vi "Insert While Loop.vi"(6 "Insertion Index":i32=-1, 7 "Parent ID":string, 8 "error in (no error)":errorcluster, 9 "Unique ID":string, 10 "Name":string, 11 "Test Executive Ref":refnum<data-value>) -> (0 "error out":errorcluster, 1 "Replaced?":bool, 3 "Test Executive Ref out":refnum<data-value>, 5 "Unique ID out":string)   [LabVIEW 2017, in "Test Executive.lvlib" / "TestExecutive Ref.lvclass"]
uses:
  <vilib>/gpm_packages/@cs/test-executive/Source/Test Executive/TestExecutive Ref/TestExecutive Ref.lvclass
  <vilib>/gpm_packages/@cs/test-executive/Source/Test Executive/ITestExecutive/ITest Executive.lvclass
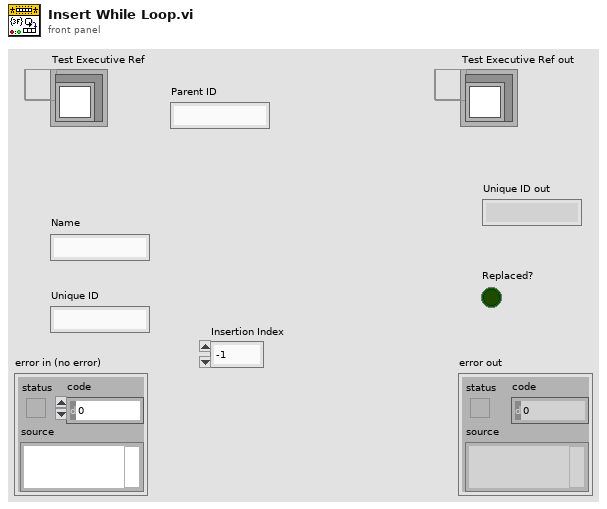
[diagram p1: front panel]
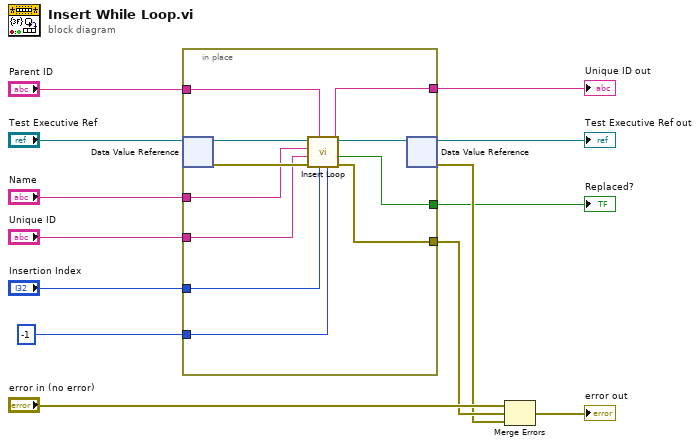
[diagram p0: block diagram]
diagram:
  n1 = in-place {
    in-place-border: "Parent ID" -> [w24]
    in-place-border: "Name" -> [w17]
    in-place-border: "Unique ID" -> [w16]
    in-place-border: "Insertion Index" -> [w22]
    in-place-border: [w23] -> w7
    in-place-border: [w21] -> w5
    in-place-border: -1 ("Loop Iterations") -> [w15]
    in-place-border: [w14] -> w1
    n2 = in-place-dvr #1("Test Executive Ref") -> (w19:refnum<class "ITest Executive.lvclass">, w18:errorcluster)
    n3 = call-dynamic "Insert Loop.vi"("Loop Iterations"=w15, "Insertion Index"=w22, "Parent ID"=w24, "error in (no error)"=w18, "Unique ID"=w16, "Name"=w17, "ITest Executive in"=w19) -> ("error out"=w21:errorcluster, "Replaced?"=w14:bool, "Unique ID out"=w23:string, "ITest Executive out"=w20:refnum<class "ITest Executive.lvclass">)  [unwired: 1 in]
    n4 = in-place-dvr #1(w20) -> (→"Test Executive Ref out":refnum<data-value>, w4:errorcluster)
  }
  "Unique ID out" <- w7
  "Replaced?" <- w1
  n5 = Merge Errors("error in (no error)", w5, w4) -> (→"error out":errorcluster)
